vi "LocalizeIOServerClassInfo.vi"(9 "Description List In":string[](array[string]), 11 "Class Names":string[](array[string])) -> (1 "Description List Out":string[](array[string]))   [LabVIEW 2017]
panel:
  in  "EPICS Client Description":string="Communicate with EPICS (Experimental Physics and Industry Control System) Servers."
  in  "Data Set Marking Description":string="Data Set Marking I/O Server allows batch logging of variable values as a set during a finite time period."
  in  "Periodic Description":string="Custom VI Server that publishes control and indicator values of the VI front panel."
  in  "On Input Change Description":string="Custom VI Server that publishes the VI input and output connection values. Values are refreshed when input value changes."
  in  "OPC Client Description":string="Communicate with OPC (OLE for Process Control) Servers."
  in  "Alarm Printer Description":string="Print alarm and event data to a line printer on a serial or parallel port."
  in  "Modbus Slave Description":string="Allow other devices or computers to read and write your data items by polling a serial port or TCP port 502 with the Modbus protocol."
  in  "Modbus Description":string="Communicate with devices that support the Modbus serial or Ethernet protocol."
  in  "EPICS Server Description":string="Publish Shared Variables to EPICS (Experimental Physics and Industrial Control System) Network."
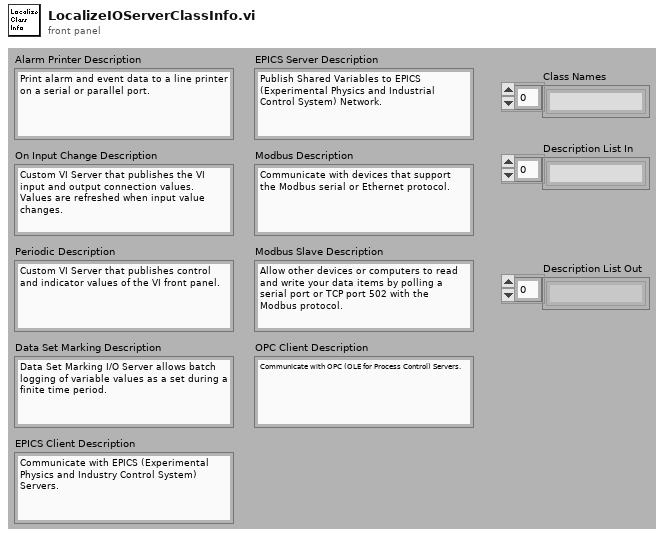
[diagram p1: front panel]
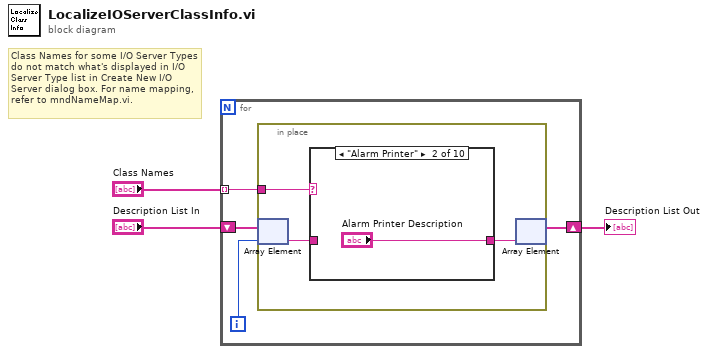
[diagram p0: block diagram]
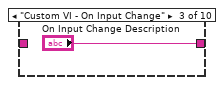
[diagram p3: hidden frame]
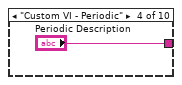
[diagram p4: hidden frame]
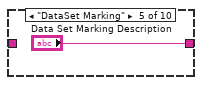
[diagram p5: hidden frame]
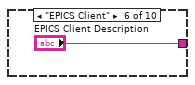
[diagram p6: hidden frame]
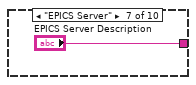
[diagram p7: hidden frame]
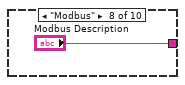
[diagram p8: hidden frame]
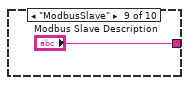
[diagram p9: hidden frame]
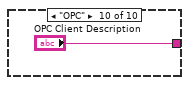
[diagram p10: hidden frame]
diagram:
  # "Class Names for some I/O Server Types do not match what's displayed in I/O Server Type list in Create New I/O Server dialog box. For name mapping, refer to mndNameMap.vi."
  n1 = for {
    tunnel: "Class Names" -> [w7] mode=indexing
    shift-right: [w5] -> w1
    shift-left: "Description List In" -> [w6]
    i -> [w4]
    n2 = in-place {
      in-place-border: w7 -> [w10]
      n3 = in-place-array #1(w6, w4) -> (w9:string)
      n4 = case shown="\"Alarm Printer\"" w10 {
        tunnel: [w11 "Alarm Printer Description" "On Input Change Description" "Periodic Description" "Data Set Marking Description" "EPICS Client Description" "EPICS Server Description" "Modbus Description" "Modbus Slave Description" "OPC Client Description"] -> w8
        tunnel: w9 -> [w11 _ _ _ _ _ _ _ _ _]
        frame Default {
        }
        frame "Alarm Printer" {
        }
        frame "Custom VI - On Input Change" {
        }
        frame "Custom VI - Periodic" {
        }
        frame "DataSet Marking" {
        }
        frame "EPICS Client" {
        }
        frame "EPICS Server" {
        }
        frame "Modbus" {
        }
        frame "ModbusSlave" {
        }
        frame "OPC" {
        }
      }
      n5 = in-place-array #1(w8) -> (w5:string[])  [unwired: 1 out]
    }
  }
  "Description List Out" <- w1
